vi "PremierVI.vi"() -> ()   [LabVIEW 2018]
panel:
  out "Gauge":dbl(knob) scale=0.0..10.0
  in  "Slide":dbl(slide) scale=0.0..10.0
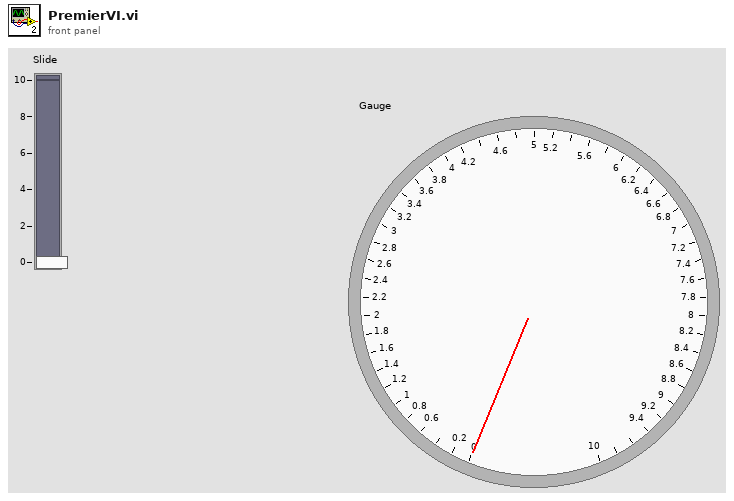
[diagram p1: front panel]
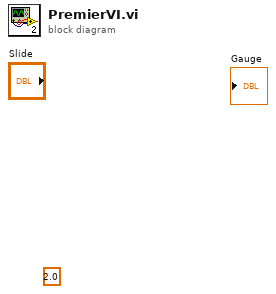
[diagram p0: block diagram]
diagram:
  (unwired) 2.0 ("y")
